vi "Adjust Text to Fit Rectangle.vi"(0 "VI Name":string, 5 "Number of Rows":i32, 7 "Text settings":T1 {"Alignment" items=["left", "center", "right"]}) -> (4 "Text out":T4)   [LabVIEW 2020, in "Text-Based VI Icon.lvlib"]
uses:
  <vilib>/LabVIEW Icon API/Set Text Icon/Text-Based VI Icon.lvlib
  <vilib>/LabVIEW Icon API/API_Text.ctl
  <vilib>/LabVIEW Icon API/API_Test Settings.ctl
  <vilib>/LabVIEW Icon API/lv_icon/Controls/Alignment.ctl
  <vilib>/LabVIEW Icon API/API_Text Colors.ctl
  13add13f-f682-447c-94c8-6f90535df557.vi
  e3a2e00b-fc37-4316-8edd-7c3cbbe33c22.vi
  Silly Billy/Exceptions.vi
  <vilib>/regexp/Match Regular Expression.xnode
  <vilib>/LabVIEW Icon API/LabVIEW Icon API.lvlib
  Silly Billy/Silly Billy.lvlib
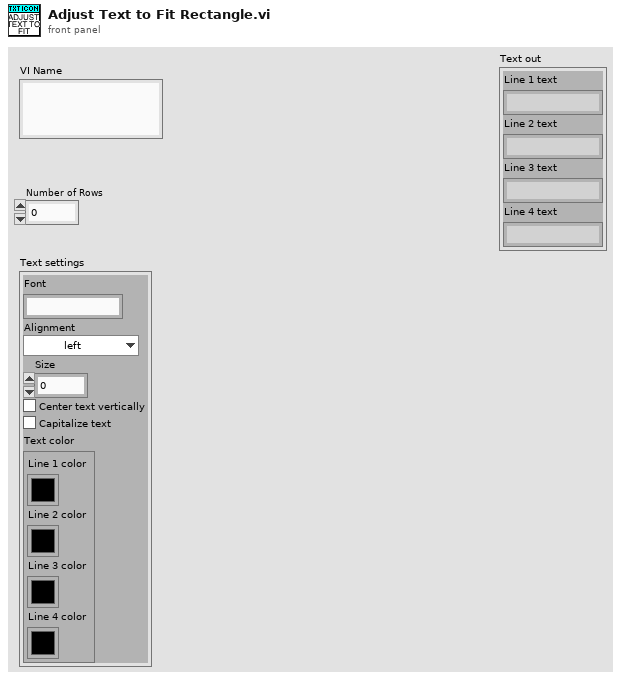
[diagram p1: front panel]
types:
  T1 = typedef "LabVIEW Icon API.lvlib/API_Test Settings.ctl" = cluster{"Font":string, "Alignment":T2, "Size":u8, "Center text":bool, "Capitalize text":bool, "Text color":T3}
  T2 = typedef "Alignment.ctl" = u16
  T3 = typedef "LabVIEW Icon API.lvlib/API_Text Colors.ctl" = cluster{"Line 1 color":u32, "Line 2 color":u32, "Line 3 color":u32, "Line 4 color":u32}
  T4 = typedef "LabVIEW Icon API.lvlib/API_Text.ctl" = cluster{"Line 1 text":string, "Line 2 text":string, "Line 3 text":string, "Line 4 text":string}
  T5 = cluster{"Font Name:":string, "Size":i16, "Strikeout?":bool, "Italic?":bool, "Underline?":bool, "Outline?":bool, "Shadow?":bool, "Bold?":bool}
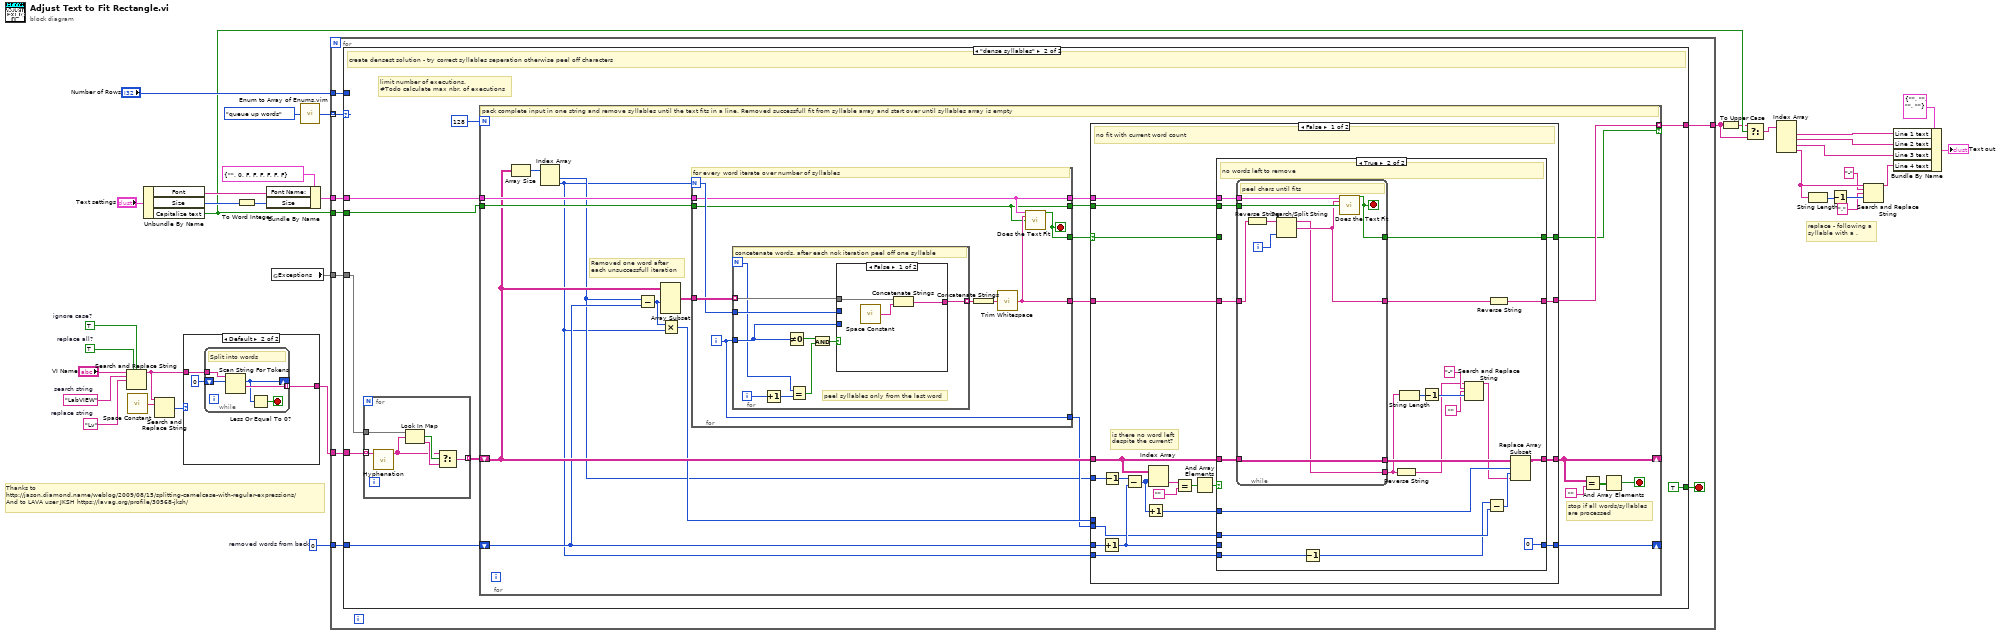
[diagram p0: block diagram]
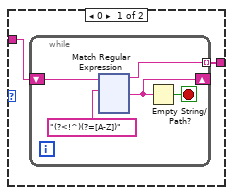
[diagram p2: hidden frame]
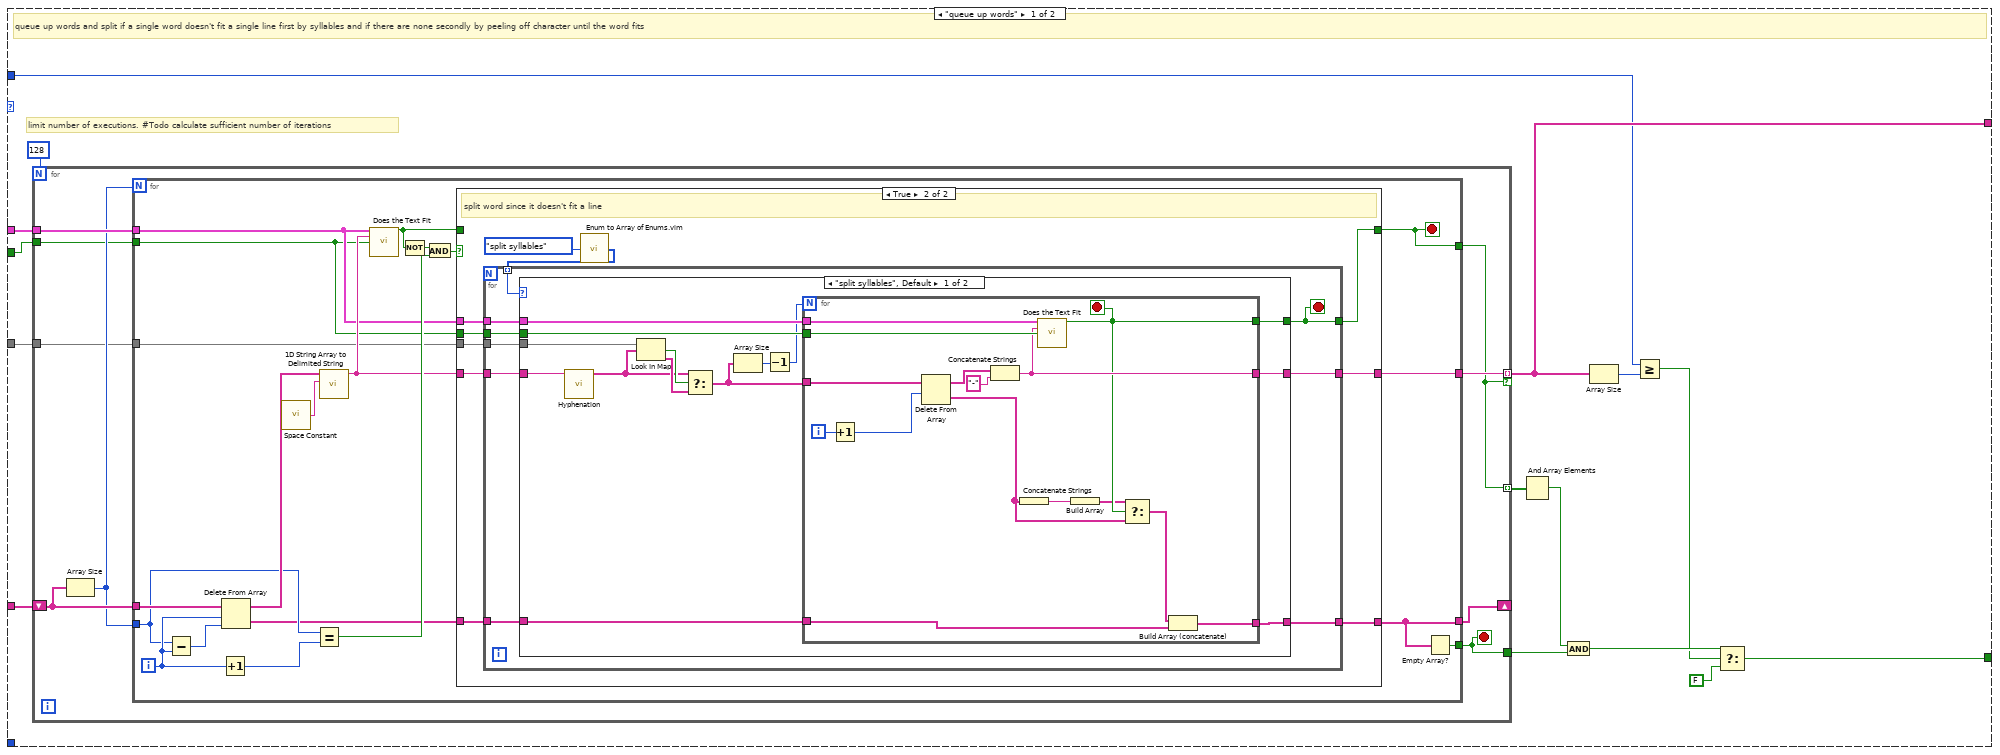
[diagram p3: hidden frame]
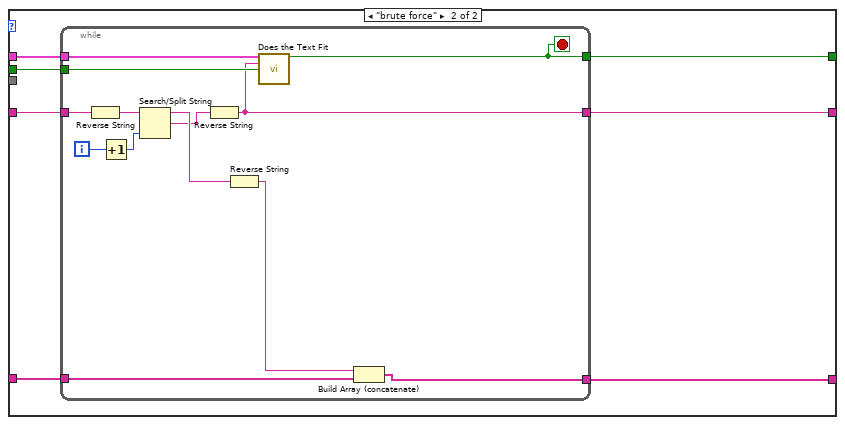
[diagram p5: hidden frame]
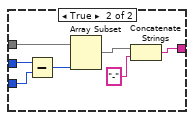
[diagram p6: hidden frame]
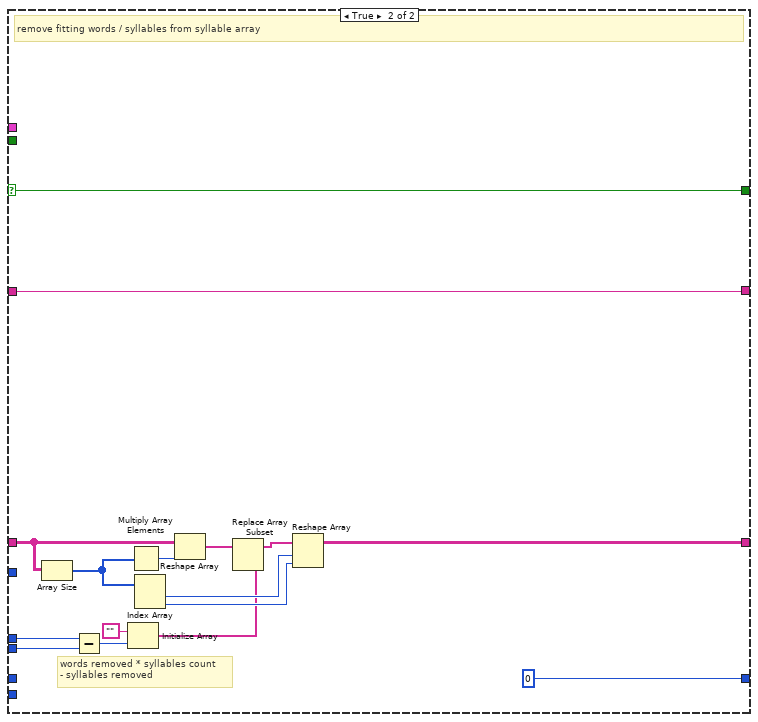
[diagram p8: hidden frame]
diagram:
  w20 = 0  # removed words from back
  w22 = TRUE  # ignore case?
  w23 = TRUE  # replace all?
  w24 = "Lv"  # replace string
  w25 = "LabVIEW"  # search string
  # "Thanks to\nhttp://jason.diamond.name/weblog/2009/08/15/splitting-camelcase-with-regular-expressions/\nAnd to LAVA user JKSH https://lavag.org/profile/30568-jksh/"
  # "replace - following a\nsyllable with a ."
  n1 = Search and Replace String(replace all?=w23, case sensitive?=w22, input string="VI Name", search string=w25, replace string=w24) -> (result string=w2:string)  [unwired: 3 in, 3 out]
  n2 = call <vilib>:"Space Constant.vi"() -> ("String"=w5:string)
  n3 = Unbundle By Name("Text settings") -> ("Font"=w29:string, "Size"=w28:u8, "Capitalize text"=w8:bool)
  n4 = Search and Replace String(input string=w2, search string=w5) -> (number of replacements=w4:i32)  [unwired: 6 in, 3 out]
  n5 = case shown="Default" w4 {
    tunnel: [w36 w159] -> w3
    tunnel: w2 -> [w37 w157]
    frame 0 {
      n6 = while {
        shift-right: [w39] -> _
        shift-left: w37 -> [w40]
        tunnel: [w38] -> w36 mode=indexing
        stop <- w42 stop-if-true
        n7 = xnode "Match Regular Expression"("input string"=w40, "regular expression"="(?<!^)(?=[A-Z])") -> ("before match"=w38:string, "after match"=w39:string)  [unwired: 4 in, 3 out]
        n8 = Empty String/Path?(string/path=w39) -> (empty?=w42:bool)
      }
    }
    frame Default {
      n9 = while {
        tunnel: w157 -> [w164]
        shift-right: [w161] -> _
        shift-left: 0 ("offset past token") -> [w163]
        tunnel: [w162] -> w159 mode=indexing
        stop <- w160 stop-if-true
        # "Split into words"
        n10 = Scan String For Tokens(8:w163, 9:w164) -> (1:w162:string, 2:w161:i32)  [unwired: 4 in, 2 out]
        n11 = Less Or Equal To 0?(x=w161) -> (x <= 0?=w160:bool)
      }
    }
  }
  n12 = To Word Integer(number=w28) -> (16bit integer=w26:i16)
  n13 = Bundle By Name(cluster=T5 {"Font Name:"="", "Size"=0, "Strikeout?"=FALSE, "Italic?"=FALSE, "Underline?"=FALSE, "Outline?"=FALSE, "Shadow?"=FALSE, "Bold?"=FALSE} ("[user-specified font]"), "Font Name:"=w29, "Size"=w26) -> (w13:T5)
  n14 = global read "Exceptions.vi" "Exceptions"() -> (w1:map{string[], string[]})
  n15 = call "Enum to Array of Enums.vim"("enum"=enum16{"queue up words", "dense syllables"}."queue up words") -> ("array of enums"=w11:enum16{"queue up words", "dense syllables"}[])
  n16 = for {
    tunnel: w8 -> [w173]
    tunnel: w20 -> [w172]
    tunnel: w13 -> [w171]
    tunnel: w11 -> [w170] mode=indexing
    tunnel: w3 -> [w169]
    tunnel: "Number of Rows" -> [w165]
    tunnel: [w167] -> w6
    tunnel: w1 -> [w166]
    stop <- w168 stop-if-true
    n17 = case shown="\"dense syllables\"" w170 {
      tunnel: [w179 w291] -> w167
      tunnel: w173 -> [w186 w297]
      tunnel: w172 -> [_ w296]
      tunnel: w171 -> [w188 w295]
      tunnel: w169 -> [w187 w293]
      tunnel: [w176 TRUE ("f")] -> w168
      tunnel: w166 -> [w180 w290]
      tunnel: w165 -> [w177 _]
      frame "queue up words" {
        # "limit number of executions. #Todo calculate sufficient number of iterations"
        # "queue up words and split if a single word doesn't fit a single line first by syllables and if there are none secondly by peeling off character until the word fits"
        n18 = for {
          N: 128 -> [_]
          tunnel: w188 -> [w197]
          tunnel: [w193] -> w179 mode=indexing if=w190
          tunnel: w186 -> [w194]
          tunnel: [w191] -> w185
          shift-right: [w192] -> _
          shift-left: w187 -> [w196]
          tunnel: [w190] -> w183 mode=indexing
          tunnel: w180 -> [w189]
          stop <- w191 stop-if-true
          n19 = Array Size(array=w196) -> (size(s)=w195:i32)
          n20 = for {
            N: w195 -> [_]
            tunnel: w197 -> [w204]
            tunnel: w196 -> [w217]
            tunnel: w195 -> [w210]
            tunnel: w194 -> [w203]
            tunnel: [w202] -> w192
            tunnel: [w199] -> w193
            tunnel: [w213] -> w191
            tunnel: [w201] -> w190
            tunnel: w189 -> [w198]
            i -> [w212]
            stop <- w201 stop-if-true
            n21 = Subtract(x=w210, y=w212) -> (x-y=w216:i32)
            n22 = Increment(x=w212) -> (x+1=w211:i32)
            n23 = Delete From Array(array=w217, length=w212, index=w216) -> (deleted portion=w205:string[], array with subset deleted=w214:string[])
            n24 = call <vilib>:"Space Constant.vi"() -> ("String"=w215:string)
            n25 = Equal?(x=w210, y=w211) -> (x = y?=w209:bool)
            n26 = call <vilib>:"1D String Array to Delimited String.vi"("delimiter"=w215, "string array"=w214) -> ("delimited string"=w206:string)  [unwired: 9 in]
            n27 = call <vilib>:"Does the Text Fit.vi"("user-specified font"=w204, "token string"=w206, "Capitalize Text"=w203) -> ("Text Fits"=w207:bool)  [unwired: 12 in]
            n28 = Not(x=w207) -> (.not. x?=w200:bool)
            n29 = And(x=w200, y=w209) -> (x .and. y?=w208:bool)
            n30 = case shown="True" w208 {
              tunnel: w207 -> [w220 _]
              tunnel: w206 -> [w218 w230]
              tunnel: w205 -> [w219 w227]
              tunnel: w204 -> [_ w226]
              tunnel: w203 -> [_ w225]
              tunnel: [w219 w224] -> w202
              tunnel: [w220 w223] -> w201
              tunnel: [w218 w222] -> w199
              tunnel: w198 -> [_ w221]
              frame False {
                # "There is a word left to remove"
              }
              frame True {
                # "split word since it doesn't fit a line"
                n31 = call "Enum to Array of Enums.vim"("enum"=enum16{"split syllables", "brute force"}."split syllables") -> ("array of enums"=w228:enum16{"split syllables", "brute force"}[])
                n32 = for {
                  tunnel: w230 -> [w239]
                  tunnel: w228 -> [w238] mode=indexing
                  tunnel: w227 -> [w237]
                  tunnel: w226 -> [w236]
                  tunnel: w225 -> [w235]
                  tunnel: [w234] -> w224
                  tunnel: [w233] -> w223
                  tunnel: [w232] -> w222
                  tunnel: w221 -> [w231]
                  stop <- w233 stop-if-true
                  n33 = case shown="\"split syllables\", Default" w238 {
                    tunnel: w239 -> [w250 w275]
                    tunnel: w237 -> [w246 w271]
                    tunnel: w236 -> [w248 w274]
                    tunnel: w235 -> [w247 w273]
                    tunnel: [w245 w270] -> w234
                    tunnel: [w244 w272] -> w233
                    tunnel: [w243 w269] -> w232
                    tunnel: w231 -> [w240 _]
                    frame "split syllables", Default {
                      n34 = call "Hyphenation.vi"("Word"=w250) -> ("Hyphenated"=w251:string[])  [unwired: 9 in, 1 out]
                      n35 = Look In Map(map=w240, key=w251) -> (key not found?=w253:bool, value=w252:string[])  [unwired: 1 in]
                      n36 = Select(t=w251, s=w253, f=w252) -> (s? t:f=w249:string[])
                      n37 = Array Size(array=w249) -> (size(s)=w242:i32)
                      n38 = Decrement(x=w242) -> (x-1=w241:i32)
                      n39 = for {
                        N: w241 -> [_]
                        tunnel: w249 -> [w268]
                        tunnel: w248 -> [w265]
                        tunnel: w247 -> [w264]
                        tunnel: w246 -> [w263]
                        tunnel: [w262] -> w245
                        tunnel: [w257] -> w244
                        tunnel: [w261] -> w243
                        i -> [w267]
                        stop <- w257 stop-if-true
                        n40 = Increment(x=w267) -> (x+1=w259:i32)
                        n41 = Delete From Array(array=w268, length=w259) -> (deleted portion=w255:string[], array with subset deleted=w266:string[])  [unwired: 1 in]
                        n42 = Concatenate Strings(w266, "-") -> (w261:string)
                        n43 = Concatenate Strings(w255) -> (w256:string)
                        n44 = call <vilib>:"Does the Text Fit.vi"("user-specified font"=w265, "token string"=w261, "Capitalize Text"=w264) -> ("Text Fits"=w257:bool)  [unwired: 12 in]
                        n45 = Build Array(w256) -> (w254:string[])
                        n46 = Select(t=w254, s=w257, f=w255) -> (s? t:f=w258:string[])
                        n47 = Build Array (concatenate)(w258, w263) -> (w262:string[])
                      }
                    }
                    frame "brute force" {
                      n48 = while {
                        tunnel: w275 -> [w288]
                        tunnel: w274 -> [w283]
                        tunnel: w273 -> [w282]
                        tunnel: [w281] -> w272
                        tunnel: w271 -> [w280]
                        tunnel: [w279] -> w270
                        tunnel: [w276] -> w269
                        i -> [w287]
                        stop <- w281 stop-if-true
                        n49 = Reverse String(1:w288) -> (0:w286:string)
                        n50 = Increment(x=w287) -> (x+1=w285:i32)
                        n51 = Search/Split String(string=w286, offset (0)=w285) -> (substring before match=w284:string, match + rest of string=w278:string)  [unwired: 1 in, 1 out]
                        n52 = Reverse String(1:w278) -> (0:w276:string)
                        n53 = Reverse String(1:w284) -> (0:w277:string)
                        n54 = call <vilib>:"Does the Text Fit.vi"("user-specified font"=w283, "token string"=w276, "Capitalize Text"=w282) -> ("Text Fits"=w281:bool)  [unwired: 12 in]
                        n55 = Build Array (concatenate)(w277, w280) -> (w279:string[])
                      }
                    }
                  }
                }
              }
            }
            n56 = Empty Array?(array=w202) -> (empty?=w213:bool)
          }
        }
        n57 = And Array Elements(Boolean array=w183) -> (logical AND=w181:bool)
        n58 = And(x=w181, y=w185) -> (x .and. y?=w182:bool)
        n59 = Array Size(array=w179) -> (size(s)=w178:i32)
        n60 = Greater Or Equal?(x=w177, y=w178) -> (x >= y?=w175:bool)
        n61 = Select(t=w182, s=w175, f=FALSE) -> (s? t:f=w176:bool)
      }
      frame "dense syllables" {
        # "limit number of executions.\n#Todo calculate max nbr. of executions"
        # "create densest solution - try correct syllables seperation otherwise peel off characters"
        n62 = for {
          tunnel: w293 -> [w303] mode=indexing
          tunnel: [w299] -> w292 mode=indexing
          tunnel: w290 -> [w298]
          n63 = call "Hyphenation.vi"("Word"=w303) -> ("Hyphenated"=w300:string[])  [unwired: 9 in, 1 out]
          n64 = Look In Map(map=w298, key=w300) -> (key not found?=w302:bool, value=w301:string[])  [unwired: 1 in]
          n65 = Select(t=w300, s=w302, f=w301) -> (s? t:f=w299:string[])
        }
        n66 = for {
          N: 128 -> [_]
          tunnel: [w308] -> w291 mode=indexing if=w305
          tunnel: w295 -> [w324]
          tunnel: w297 -> [w323]
          shift-right: [w321] -> _
          shift-left: w292 -> [w322]
          shift-right: [w314] -> _
          shift-left: w296 -> [w311]
          stop <- w312 stop-if-true
          # "stop if all words/syllables\nare processed"
          # "Removed one word after\neach unsuccessfull iteration"
          # "pack complete input in one string and remove syllables until the text fits in a line. Removed successfull fit from syllable array and start over until syllables array is empty"
          n67 = Array Size(array=w322) -> (size(s)=w325:i32[])
          n68 = Index Array(array=w325) -> (element #1=w310:i32, element #2=w304:i32)  [unwired: 2 in]
          n69 = Subtract(x=w310, y=w311) -> (x-y=w317:i32)
          n70 = Array Subset(array=w322, length (row)=w317) -> (w318:string[][])  [unwired: 3 in]
          n71 = Multiply(x=w317, y=w304) -> (x*y=w316:i32)
          n72 = for {
            N: w304 -> [w330]
            tunnel: [w332] -> w309
            tunnel: w318 -> [w334]
            tunnel: w324 -> [w328]
            tunnel: w323 -> [w327]
            tunnel: [w331] -> w313
            tunnel: [w329] -> w315
            tunnel: [w328] -> w307
            tunnel: [w327] -> w306
            i -> [w329]
            stop <- w331 stop-if-true
            # "for every word iterate over number of syllables"
            n73 = for {
              N -> [w338]
              tunnel: [w344] -> w333 mode=indexing
              tunnel: w330 -> [w343]
              tunnel: w329 -> [w342]
              tunnel: w334 -> [w341] mode=indexing
              i -> [w336]
              # "peel syllables only from the last word"
              # "concetenate words. after each nok iteration peel off one syllable"
              n74 = Increment(x=w336) -> (x+1=w339:i32)
              n75 = Not Equal To 0?(x=w342) -> (x != 0?=w335:bool)
              n76 = Equal?(x=w338, y=w339) -> (x = y?=w337:bool)
              n77 = And(x=w335, y=w337) -> (x .and. y?=w340:bool)
              n78 = case shown="False" w340 {
                tunnel: [w347 w354] -> w344
                tunnel: w341 -> [w346 w352]
                tunnel: w342 -> [_ w351]
                tunnel: w343 -> [_ w350]
                frame False {
                  n79 = call <vilib>:"Space Constant.vi"() -> ("String"=w345:string)
                  n80 = Concatenate Strings(w346, w345) -> (w347:string)
                }
                frame True {
                  n81 = Subtract(x=w350, y=w351) -> (x-y=w348:i32)
                  n82 = Array Subset(array=w352, length=w348) -> (w353:string[])  [unwired: 1 in]
                  n83 = Concatenate Strings(w353, "-") -> (w354:string)
                }
              }
            }
            n84 = Concatenate Strings(w333) -> (w326:string)
            n85 = call <vilib>:"Trim Whitespace.vi"("string"=w326) -> ("trimmed string"=w332:string)  [unwired: 1 in]
            n86 = call <vilib>:"Does the Text Fit.vi"("user-specified font"=w328, "token string"=w332, "Capitalize Text"=w327) -> ("Text Fits"=w331:bool)  [unwired: 12 in]
          }
          n87 = case shown="False" w313 {
            selector: w313 -> [w364 w411]
            tunnel: w322 -> [w369 w426]
            tunnel: [w371 w419] -> w321
            tunnel: w316 -> [_ w420]
            tunnel: w315 -> [w360 w421]
            tunnel: w311 -> [w375 _]
            tunnel: [w367 0] -> w314
            tunnel: w310 -> [w357 _]
            tunnel: w309 -> [w373 w412]
            tunnel: [w372 w412] -> w308
            tunnel: w307 -> [w374 _]
            tunnel: w306 -> [w370 _]
            tunnel: [w363 w411] -> w305
            tunnel: w304 -> [w361 _]
            frame False {
              # "is there no word left\ndespite the current?"
              # "no fit with current word count"
              n88 = Increment(x=w375) -> (x+1=w368:i32)
              n89 = Decrement(x=w357) -> (x-1=w362:i32)
              n90 = Subtract(x=w362, y=w368) -> (x-y=w356:i32)
              n91 = Increment(x=w356) -> (x+1=w355:i32)
              n92 = Index Array(array=w369, index (row)=w356) -> (element=w359:string[])  [unwired: 1 in]
              n93 = Equal?(x=w359, y="") -> (x = y?=w365:bool[])
              n94 = And Array Elements(Boolean array=w365) -> (logical AND=w358:bool)
              n95 = case shown="True" w358 {
                tunnel: w374 -> [_ w401]
                tunnel: w373 -> [w379 w400]
                tunnel: [w379 w387] -> w372
                tunnel: w369 -> [w378 w392]
                tunnel: [w378 w394] -> w371
                tunnel: w370 -> [_ w398]
                tunnel: w368 -> [w377 _]
                tunnel: [w377 0] -> w367
                tunnel: w364 -> [w376 _]
                tunnel: [w376 w396] -> w363
                tunnel: w355 -> [_ w393]
                tunnel: w361 -> [_ w391]
                tunnel: w360 -> [_ w390]
                frame False {
                  # "remove a word for next fit check"
                }
                frame True {
                  # "no words left to remove"
                  n96 = while {
                    tunnel: w401 -> [w410]
                    tunnel: w400 -> [w409]
                    tunnel: [w405] -> w399
                    tunnel: w392 -> [w403]
                    tunnel: w398 -> [w406]
                    tunnel: [w402] -> w381
                    tunnel: [w404] -> w396
                    tunnel: [w403] -> w395
                    i -> [w407]
                    stop <- w404 stop-if-true
                    # "peel chars until fits"
                    n97 = Reverse String(1:w409) -> (0:w408:string)
                    n98 = Search/Split String(string=w408, offset (0)=w407) -> (substring before match=w402:string, match + rest of string=w405:string)  [unwired: 1 in, 1 out]
                    n99 = call <vilib>:"Does the Text Fit.vi"("user-specified font"=w410, "token string"=w405, "Capitalize Text"=w406) -> ("Text Fits"=w404:bool)  [unwired: 12 in]
                  }
                  n100 = Decrement(x=w391) -> (x-1=w388:i32)
                  n101 = Reverse String(1:w381) -> (0:w382:string)
                  n102 = String Length(string=w381) -> (length=w385:i32)
                  n103 = Decrement(x=w385) -> (x-1=w386:i32)
                  n104 = Search and Replace String(input string=w382, search string="-", replace string="" ("replace string (\"\")"), offset=w386) -> (result string=w380:string)  [unwired: 4 in, 3 out]
                  n105 = Subtract(x=w388, y=w390) -> (x-y=w389:i32)
                  n106 = Reverse String(1:w399) -> (0:w387:string)
                  n107 = Replace Array Subset(array=w395, new element=w380, index (row)=w393, index (col)=w389) -> (w394:string[][])
                }
              }
            }
            frame True {
              # "words removed * syllables count\n- syllables removed"
              # "remove fitting words / syllables from syllable array"
              n108 = Array Size(array=w426) -> (size(s)=w425:i32[])
              n109 = Subtract(x=w420, y=w421) -> (x-y=w416:i32)
              n110 = Initialize Array("", w416) -> (w414:string[])
              n111 = Multiply Array Elements(1:w425) -> (0:w422:i32)
              n112 = Index Array(array=w425) -> (element #1=w418:i32, element #2=w417:i32)  [unwired: 2 in]
              n113 = Reshape Array(w426, w422) -> (w424:string[])
              n114 = Replace Array Subset(array=w424, new element=w414) -> (w423:string[])  [unwired: 1 in]
              n115 = Reshape Array(w423, w418, w417) -> (w419:string[][])
            }
          }
          n116 = Equal?(x=w321, y="") -> (x = y?=w319:bool[][])
          n117 = And Array Elements(Boolean array=w319) -> (logical AND=w312:bool)
        }
      }
    }
  }
  n118 = To Upper Case(1:w6) -> (0:w7:string[])
  n119 = Select(t=w7, s=w8, f=w6) -> (s? t:f=w9:string[])
  n120 = Index Array(array=w9) -> (element #1=w32:string, element #2=w33:string, element #3=w34:string, element #4=w17:string)  [unwired: 4 in]
  n121 = String Length(string=w17) -> (length=w19:i32)
  n122 = Decrement(x=w19) -> (x-1=w18:i32)
  n123 = Search and Replace String(input string=w17, search string="-", replace string="." ("replace string (\"\")"), offset=w18) -> (result string=w14:string)  [unwired: 4 in, 3 out]
  n124 = Bundle By Name(cluster=T4 {"Line 1 text"="", "Line 2 text"="", "Line 3 text"="", "Line 4 text"=""} ("Text out"), "Line 1 text"=w32, "Line 2 text"=w33, "Line 3 text"=w34, "Line 4 text"=w14) -> (→"Text out":T4)
